vi "BitTest.vi"(7 "error in (no error)":errorcluster, 8 "BitAddr":u32, 9 "Offset":u32) -> (0 "error out":errorcluster, 2 "Bool Board 2":bool, 3 "Bool Board 1":bool)   [LabVIEW 2015, in "ESLSCDLL.lvlib"]
uses:
  ESLSCDLL.lvlib
  Globals.vi
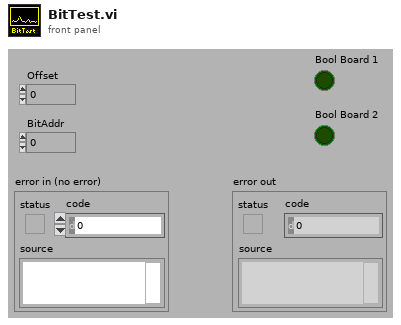
[diagram p1: front panel]
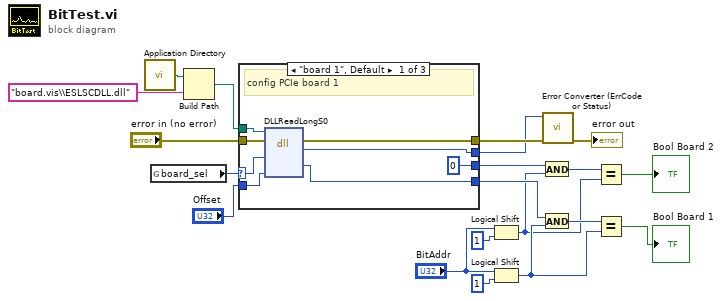
[diagram p0: block diagram]
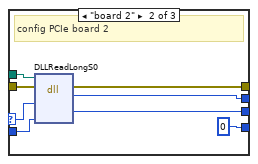
[diagram p2: hidden frame]
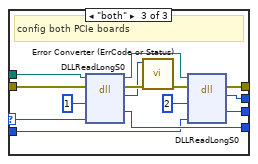
[diagram p3: hidden frame]
diagram:
  n1 = call <vilib>:"Application Directory.vi"() -> ("Application Directory"=w3:path)
  n2 = global read "Globals.vi" "board_sel"() -> (w4:enum32{"0", "board 1", "board 2", "both"})
  n3 = Build Path(base path=w3, name or relative path="board.vis\\ESLSCDLL.dll") -> (appended path=w1:path)
  n4 = case shown="\"board 1\", Default" w4 {
    selector: w4 -> [w26 w35 w45]
    tunnel: [w28 u32 0 w50] -> w18
    tunnel: "Offset" -> [w27 w34 w48]
    tunnel: [u32 0 w36 w49] -> w11
    tunnel: "error in (no error)" -> [w24 w32 w44]
    tunnel: [w23 w30 w40] -> w7
    tunnel: [w22 w31 w39] -> w6
    tunnel: w1 -> [w21 w29 w38]
    frame "board 1", Default {
      # "config PCIe board 1"
      n5 = dll-call lib="C:/ENTW/PCIE/LV64/board.vis/ESLSCDLL.dll" fn="DLLReadLongS0"(path in=w21, error in=w24, "drv"=w26, "PortOff"=w27) -> (error out=w23:errorcluster, "es_status_codes"=w22:i32, "data"=w28:u32)  [unwired: 4 in, 1 out]
    }
    frame "board 2" {
      # "config PCIe board 2"
      n6 = dll-call lib="C:/ENTW/PCIE/LV64/board.vis/ESLSCDLL.dll" fn="DLLReadLongS0"(path in=w29, error in=w32, "drv"=w35, "PortOff"=w34) -> (error out=w30:errorcluster, "es_status_codes"=w31:i32, "data"=w36:u32)  [unwired: 4 in, 1 out]
    }
    frame "both" {
      # "config both PCIe boards"
      n7 = dll-call lib="C:/ENTW/PCIE/LV64/board.vis/ESLSCDLL.dll" fn="DLLReadLongS0"(path in=w38, error in=w44, "drv"=u32 1, "PortOff"=w45) -> (path out=w37:path, error out=w43:errorcluster, "es_status_codes"=w42:i32, "data"=w50:u32)  [unwired: 4 in]
      n8 = call "Error Converter (ErrCode or Status).vi"("error in (no error)"=w43, "error code"=w42) -> ("error out"=w41:errorcluster)  [unwired: 9 in]
      n9 = dll-call lib="C:/ENTW/PCIE/LV64/board.vis/ESLSCDLL.dll" fn="DLLReadLongS0"(path in=w37, error in=w41, "drv"=u32 2, "PortOff"=w48) -> (error out=w40:errorcluster, "es_status_codes"=w39:i32, "data"=w49:u32)  [unwired: 4 in, 1 out]
    }
  }
  n10 = Logical Shift(y="BitAddr", x=u32 1) -> (x << y=w13:u32)
  n11 = Logical Shift(y="BitAddr", x=u32 1) -> (x << y=w16:u32)
  n12 = And(x=w11, y=w13) -> (x .and. y?=w12:u32)
  n13 = And(x=w18, y=w16) -> (x .and. y?=w19:u32)
  n14 = call "Error Converter (ErrCode or Status).vi"("error in (no error)"=w7, "error code"=w6) -> ("error out"=→"error out":errorcluster)  [unwired: 9 in]
  n15 = Equal?(x=w12, y=w13) -> (x = y?=→"Bool Board 2":bool)
  n16 = Equal?(x=w19, y=w16) -> (x = y?=→"Bool Board 1":bool)
